vi "Control - FuelSplitNormalizer.vi"(7 "Fuel Splits []":sgl[](array[numeric])) -> (8 "Normalized Fuel Splits [Frac]":sgl[](array[numeric]))   [LabVIEW 2015, in "ECS-RT.lvlib"]
uses:
  ECS-RT.lvlib
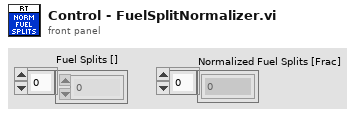
[diagram p1: front panel]
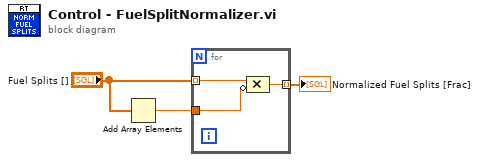
[diagram p0: block diagram]
diagram:
  n1 = Add Array Elements(numeric array="Fuel Splits []") -> (sum=w2:sgl)
  n2 = for {
    tunnel: "Fuel Splits []" -> [w4] mode=indexing
    tunnel: w2 -> [w6]
    tunnel: [w5] -> w1 mode=indexing
    n3 = Compound Arithmetic op=MULTIPLY(w4, invert w6) -> (w5:sgl)
  }
  "Normalized Fuel Splits [Frac]" <- w1
